vi "MTS_IntensityArrayToImage.vi"(0 "Image":T1, 1 "Image":i32[][](array[numeric]), 11 "error in (no error)":errorcluster, 12 "Log Scale":bool) -> (4 "Image Out":T1, 15 "error out":errorcluster)   [LabVIEW 2011]
uses:
  <vilib>/vision/Image Controls.llb/IMAQ Image.ctl
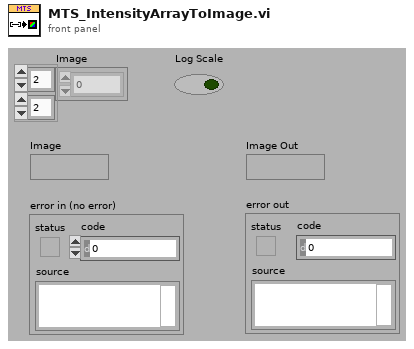
[diagram p1: front panel]
types:
  T1 = typedef "IMAQ Image.ctl" = refnum<image>
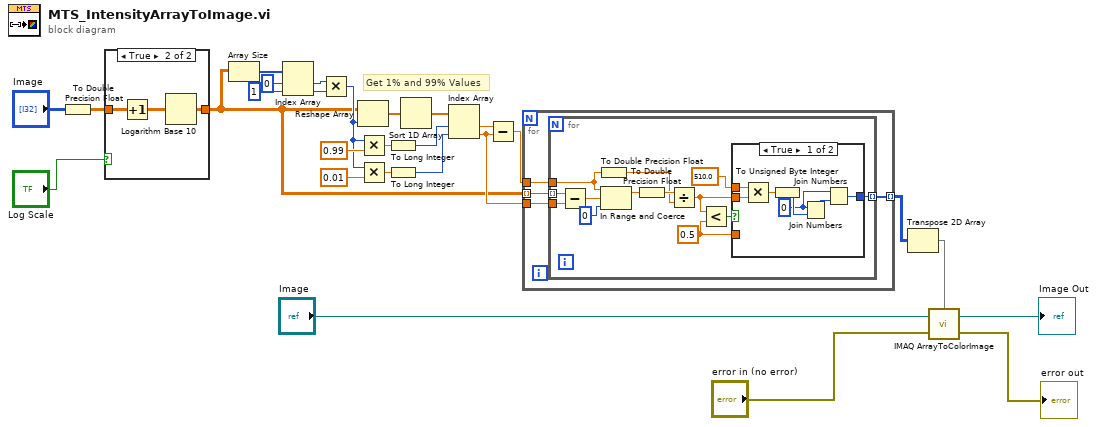
[diagram p0: block diagram]
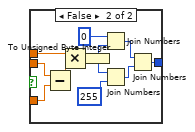
[diagram p3: hidden frame]
diagram:
  # "Get 1% and 99% Values"
  n1 = To Double Precision Float(number="Image") -> (double precision float=w3:dbl[][])
  n2 = case shown="True" "Log Scale" {
    tunnel: w3 -> [w28 w30]
    tunnel: [w28 w31] -> w2
    frame False {
    }
    frame True {
      n3 = Increment(x=w30) -> (x+1=w29:dbl[][])
      n4 = Logarithm Base 10(1:w29) -> (0:w31:dbl[][])
    }
  }
  n5 = Array Size(array=w2) -> (size(s)=w6:i32[])
  n6 = Index Array(array=w6, index #1=0 ("index"), index #2=1 ("index")) -> (element #1=w9:i32, element #2=w10:i32)
  n7 = Multiply(x=w9, y=w10) -> (x*y=w13:i32)
  n8 = Reshape Array(w2, w13) -> (w11:dbl[])
  n9 = Multiply(x=w13, y=0.99) -> (x*y=w16:dbl)
  n10 = Multiply(x=w13, y=0.01) -> (x*y=w17:dbl)
  n11 = To Long Integer(number=w16) -> (32bit integer=w19:i32)
  n12 = To Long Integer(number=w17) -> (32bit integer=w18:i32)
  n13 = Sort 1D Array(array=w11) -> (sorted array=w12:dbl[])
  n14 = Index Array(array=w12, index #1=w19, index #2=w18) -> (element #1=w20:dbl, element #2=w21:dbl)
  n15 = Subtract(x=w20, y=w21) -> (x-y=w22:dbl)
  n16 = for {
    tunnel: w2 -> [w35] mode=indexing
    tunnel: w21 -> [w34]
    tunnel: w22 -> [w33]
    tunnel: [w32] -> w27 mode=indexing
    n17 = for {
      tunnel: w35 -> [w48] mode=indexing
      tunnel: w34 -> [w47]
      tunnel: w33 -> [w43]
      tunnel: [w37] -> w32 mode=indexing
      w36 = 0.5 ("y")
      n18 = Subtract(x=w48, y=w47) -> (x-y=w46:dbl)
      n19 = To Double Precision Float(number=w43) -> (double precision float=w41:dbl)
      n20 = In Range and Coerce(upper limit=w43, x=w46, lower limit=0) -> (coerced(x)=w44:dbl)  [unwired: 1 out]
      n21 = To Double Precision Float(number=w44) -> (double precision float=w42:dbl)
      n22 = Divide(x=w42, y=w41) -> (x/y=w39:dbl)
      n23 = Less?(x=w39, y=w36) -> (x < y?=w40:bool)
      n24 = case shown="True" w40 {
        tunnel: w39 -> [w55 w62]
        tunnel: 510.0 ("y") -> [w54 w66]
        tunnel: [w50 w63] -> w37
        tunnel: w36 -> [_ w61]
        frame True {
          w49 = u8 0 ("hi")
          n25 = Multiply(x=w54, y=w55) -> (x*y=w53:dbl)
          n26 = To Unsigned Byte Integer(number=w53) -> (unsigned 8bit integer=w51:u8)
          n27 = Join Numbers(hi=w49, lo=w51) -> ((hi.lo)=w52:u16)
          n28 = Join Numbers(hi=w49, lo=w52) -> ((hi.lo)=w50:u32)
        }
        frame False {
          n29 = Subtract(x=w62, y=w61) -> (x-y=w60:dbl)
          n30 = Multiply(x=w66, y=w60) -> (x*y=w65:dbl)
          n31 = To Unsigned Byte Integer(number=w65) -> (unsigned 8bit integer=w59:u8)
          n32 = Join Numbers(hi=u8 0, lo=w59) -> ((hi.lo)=w58:u16)
          n33 = Join Numbers(hi=w59, lo=u8 255) -> ((hi.lo)=w64:u16)
          n34 = Join Numbers(hi=w58, lo=w64) -> ((hi.lo)=w63:u32)
        }
      }
    }
  }
  n35 = Transpose 2D Array(2D array=w27) -> (transposed array=w1:u32[][])
  n36 = call "IMAQ ArrayToColorImage"("Image Pixels (U32)"=w1, "Image"="Image", "error in (no error)"="error in (no error)") -> ("Image Out"=→"Image Out":T1, "error out"=→"error out":errorcluster)  [unwired: 2 in]
